vi "Report.vi"() -> ()   [LabVIEW 2017]
uses:
  <vilib>/Utility/miscctls.llb/LVRowAndColumnUnsignedTypeDef.ctl
  bcf87072-937c-4590-92ea-1cc62e0fba93.vi
  a160b8e7-0040-4e34-a052-5f80b3aab475.vi
  <vilib>/Array/Sort 2D Array - Pop Stack.vi
  <vilib>/Array/Sort 2D Array - Push Stack.vi
  <vilib>/addons/database/Connection.llb/DB Tools Open Connec (String).vi
  <vilib>/Utility/file.llb/Write Delimited Spreadsheet (string).vi
  Global/Global 1.vi
  <vilib>/regexp/Match Regular Expression.xnode
  <vilib>/addons/database/NI_Database_API.lvlib
  <vilib>/Utility/NIReport.llb/NI_report.lvclass
  <vilib>/Utility/NIReport.llb/Append Text Table to Report (wrap).vi
panel:
  out "reposr save header":string[](array[string])
  in  "SELECT REPORT TYPE":string(combo)="WITH TRECIABILITY"
  out "error out":errorcluster
  in  "error in (no error)":errorcluster
  in  "GET REPORT":bool
  in  "EXIT":bool
  in  "EXPORT TO EXCEL":bool
  in  "TO":timestamp format="%<%x>T"
  in  "FROM":timestamp format="%<%x>T"
  in  "BARCODE":string
  in  "TYPE":string(combo)="DATE TIME"
  in  "STATION WISE":string(combo)="0"
  out "Table":string[][](table)
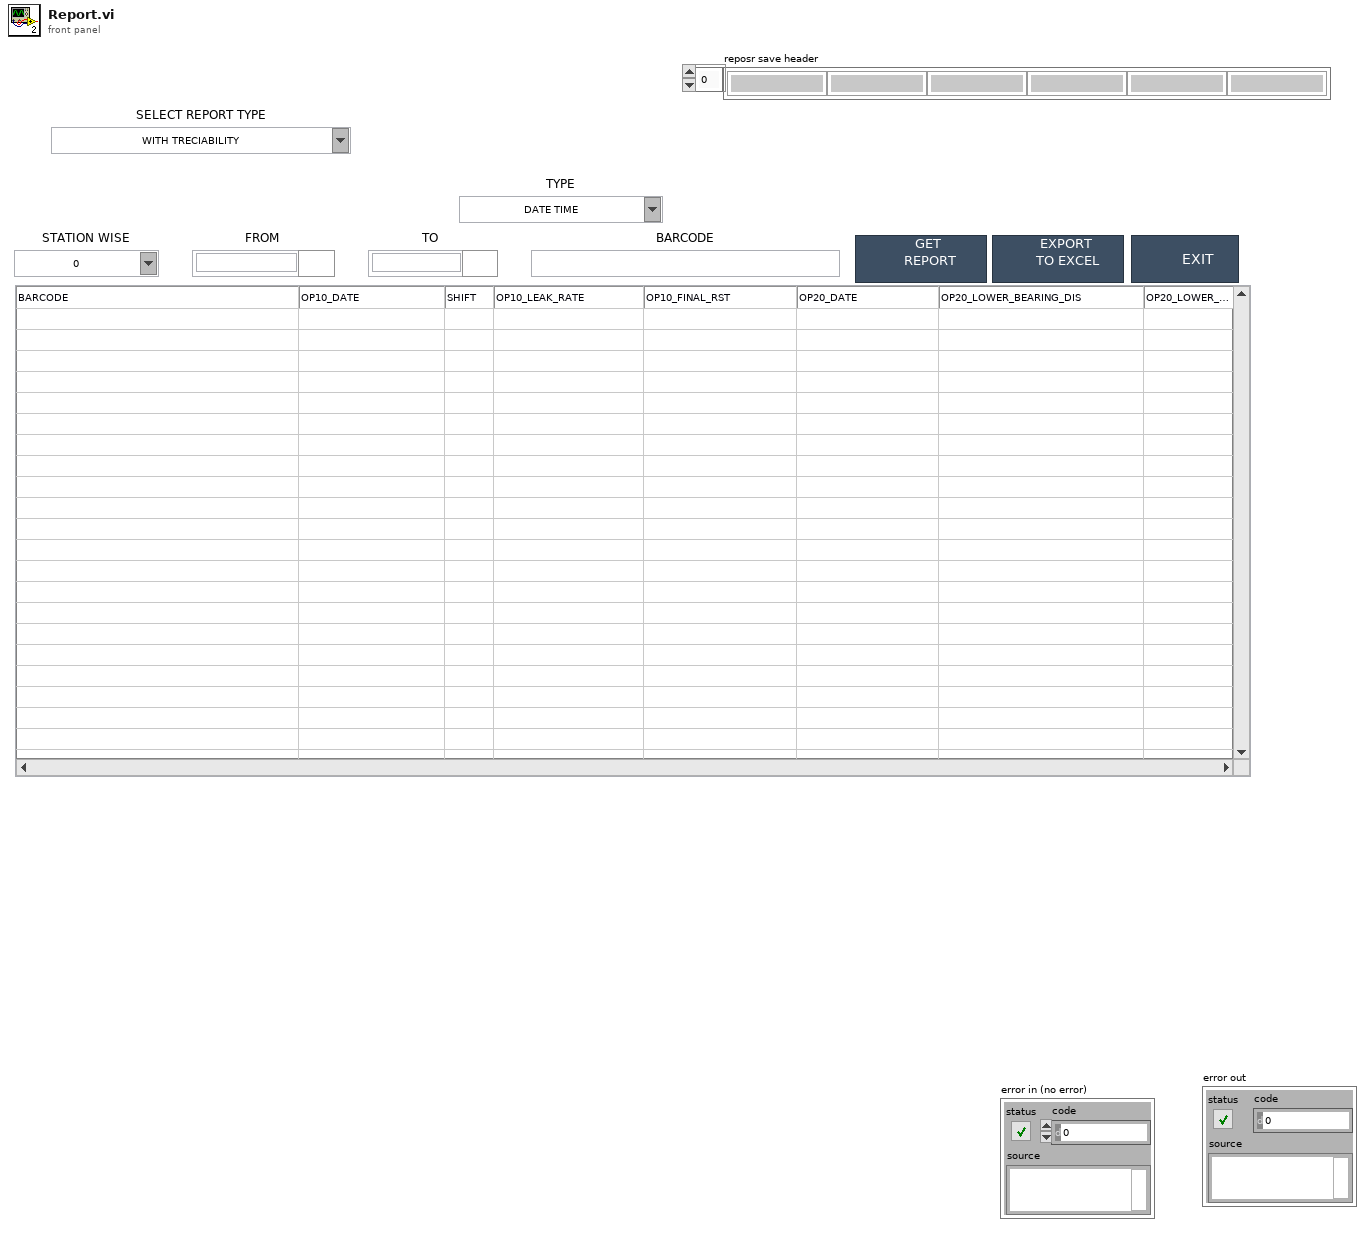
[diagram p1: front panel]
types:
  T1 = typedef "NI_Database_API.lvlib/Conn ObjectReference.ctl" = refnum<k1>
  T2 = typedef "LVRowAndColumnUnsignedTypeDef.ctl" = cluster{"Row":u32, "Column":u32}
  T3 = enum16{"Standard Report", "HTML", "Word", "Excel"}
  T4 = enum16{"maximized", "minimized", "normal", "no change"}
  T5 = typedef "LVRowAndColumnTypeDef.ctl" = cluster{"Row":i32, "Column":i32}
  T6 = enum32{"invalid app kind", "Development System", "Run Time System", "Student Edition", "Embedded LabVIEW", "Evaluation", "Custom"}
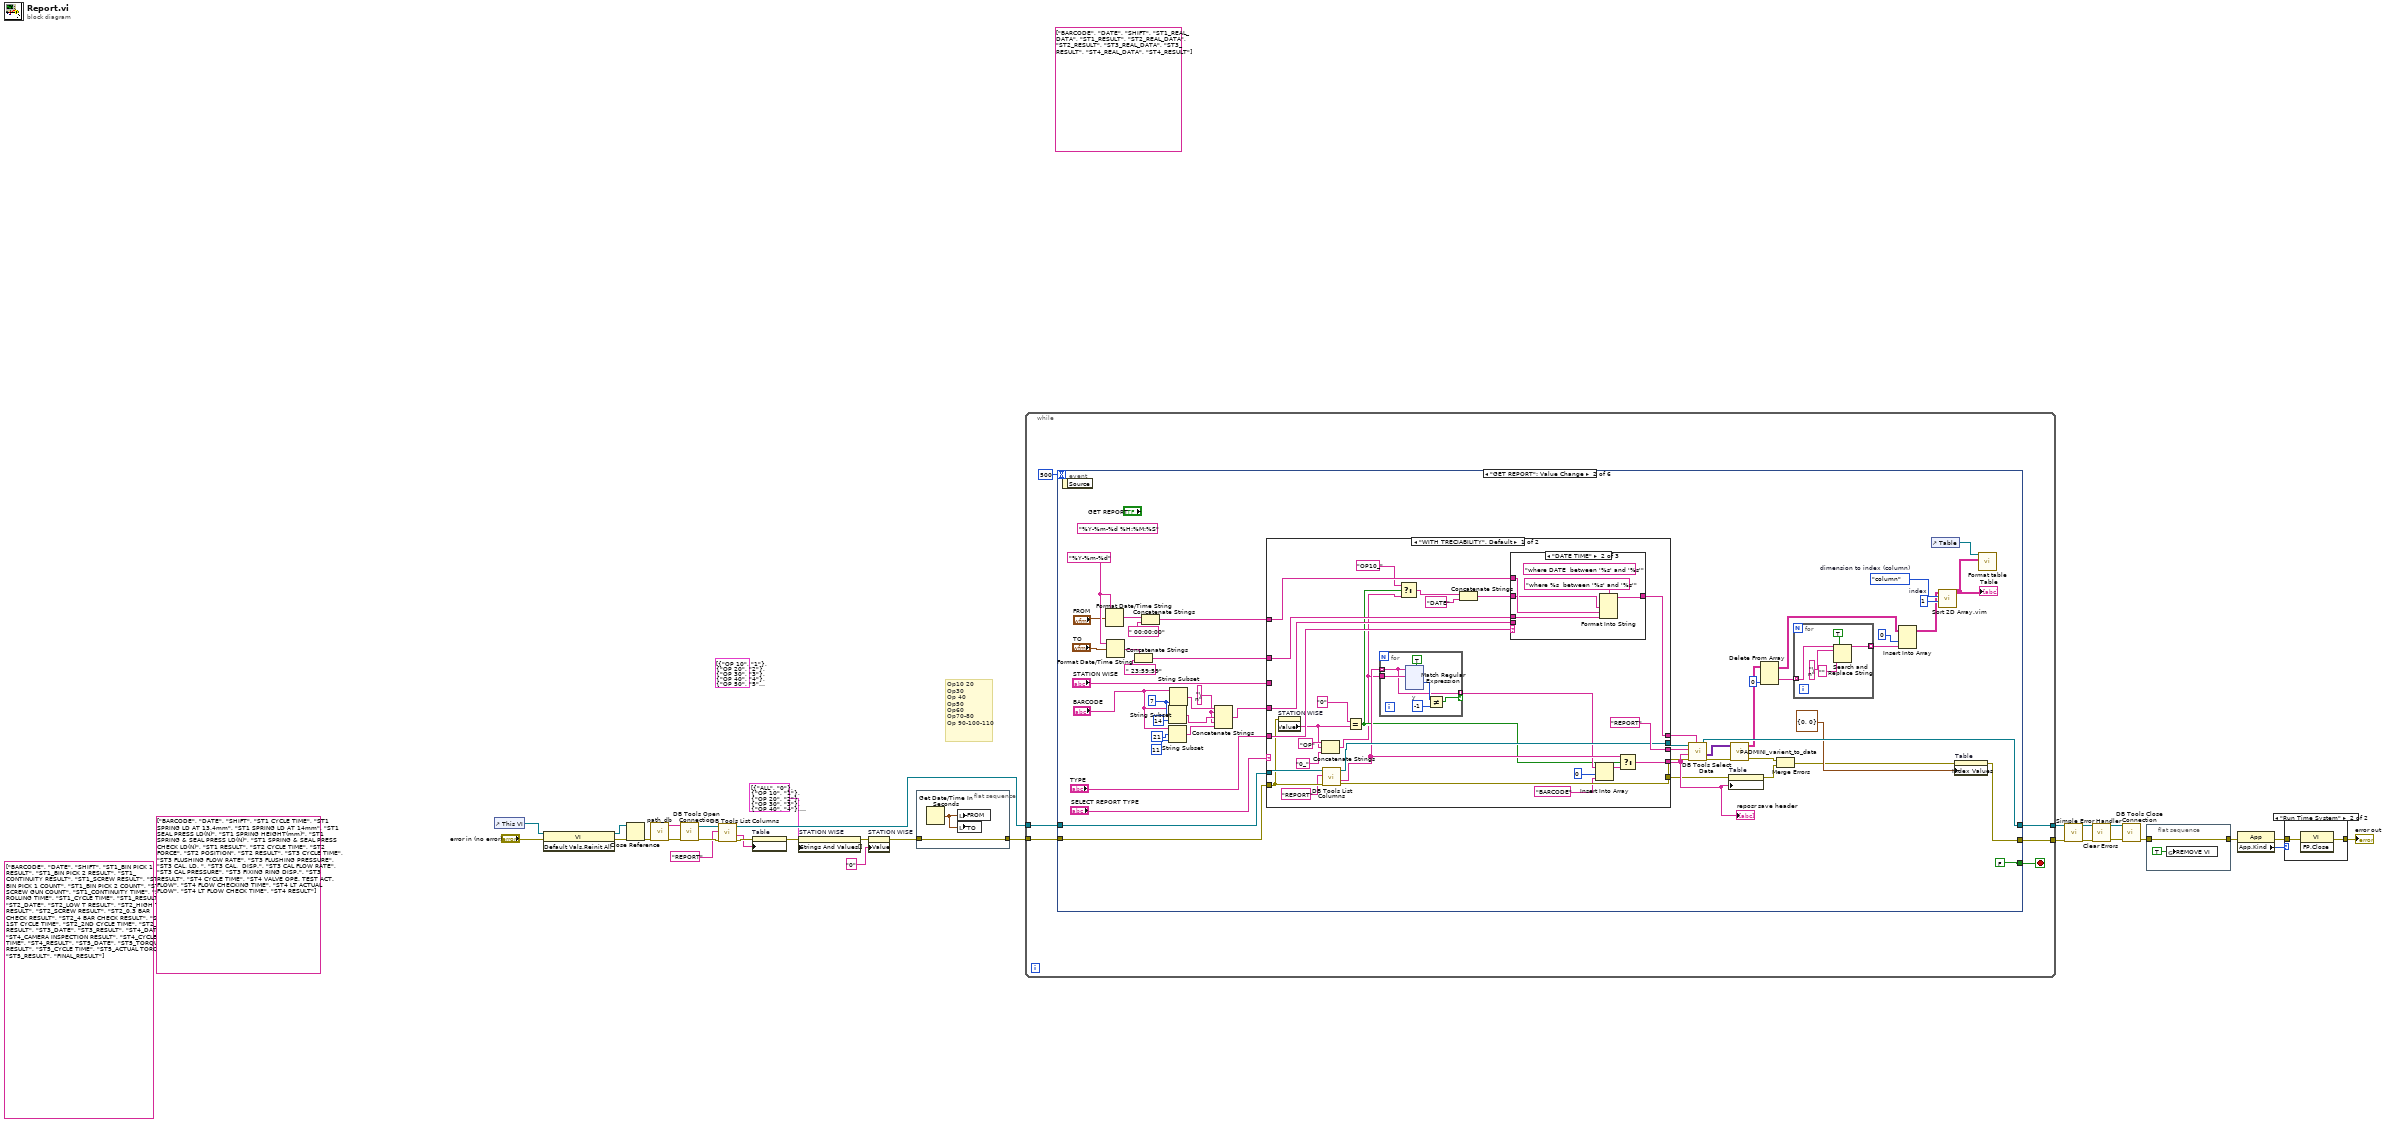
[diagram p0: block diagram]
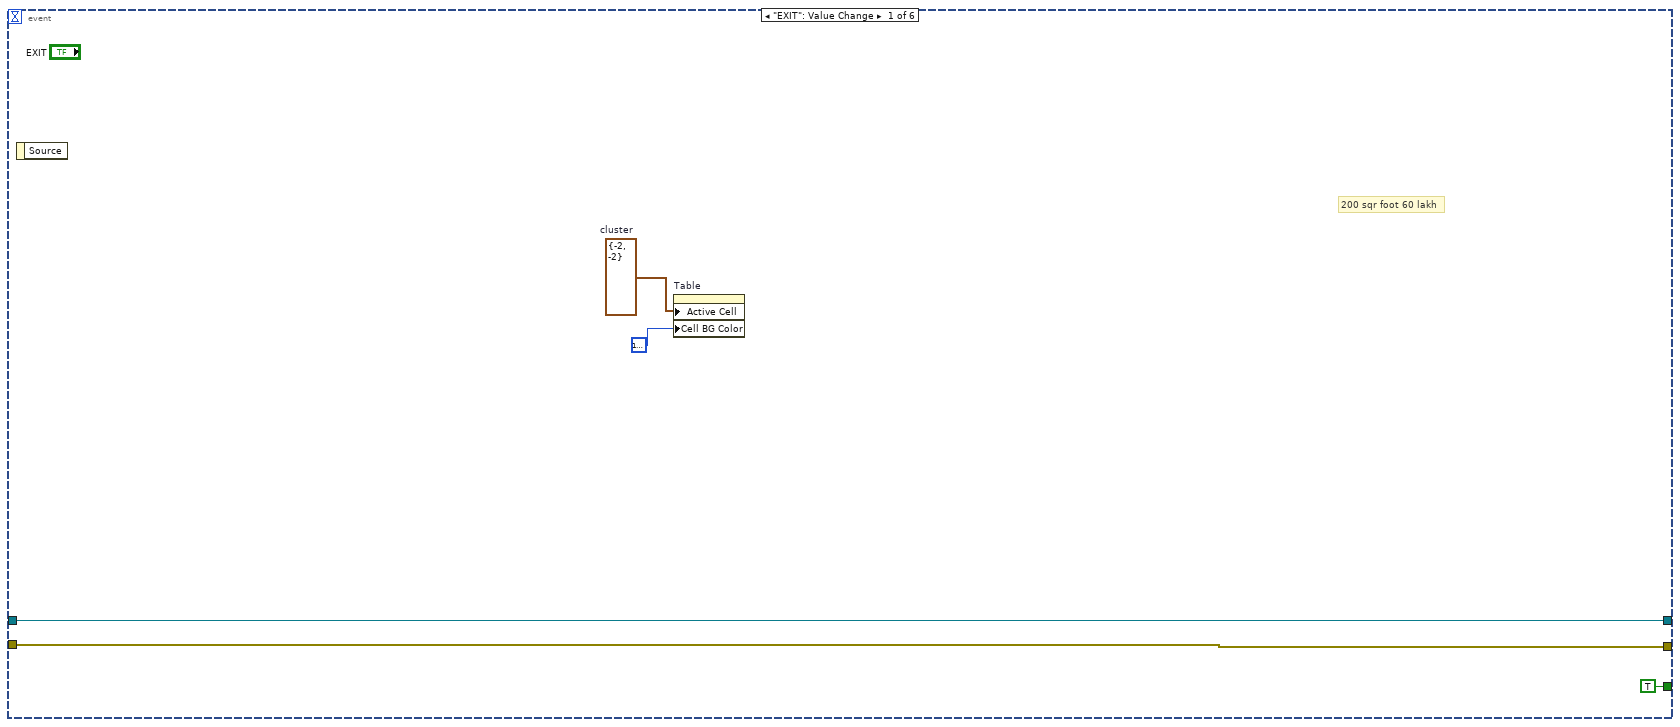
[diagram p2: hidden frame]
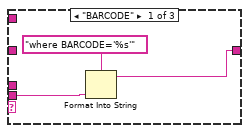
[diagram p3: hidden frame]
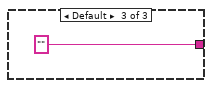
[diagram p4: hidden frame]
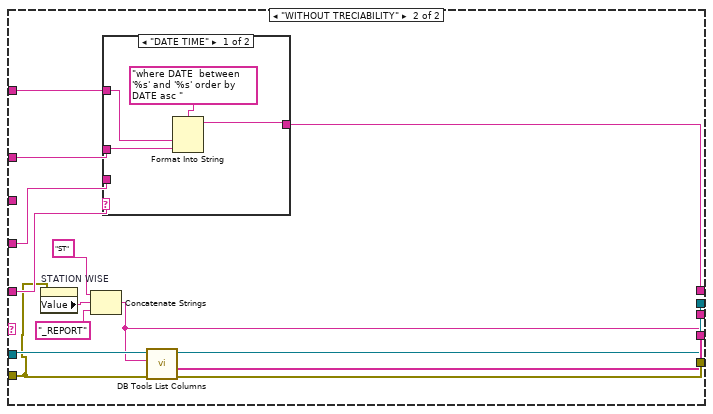
[diagram p5: hidden frame]
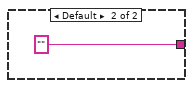
[diagram p6: hidden frame]
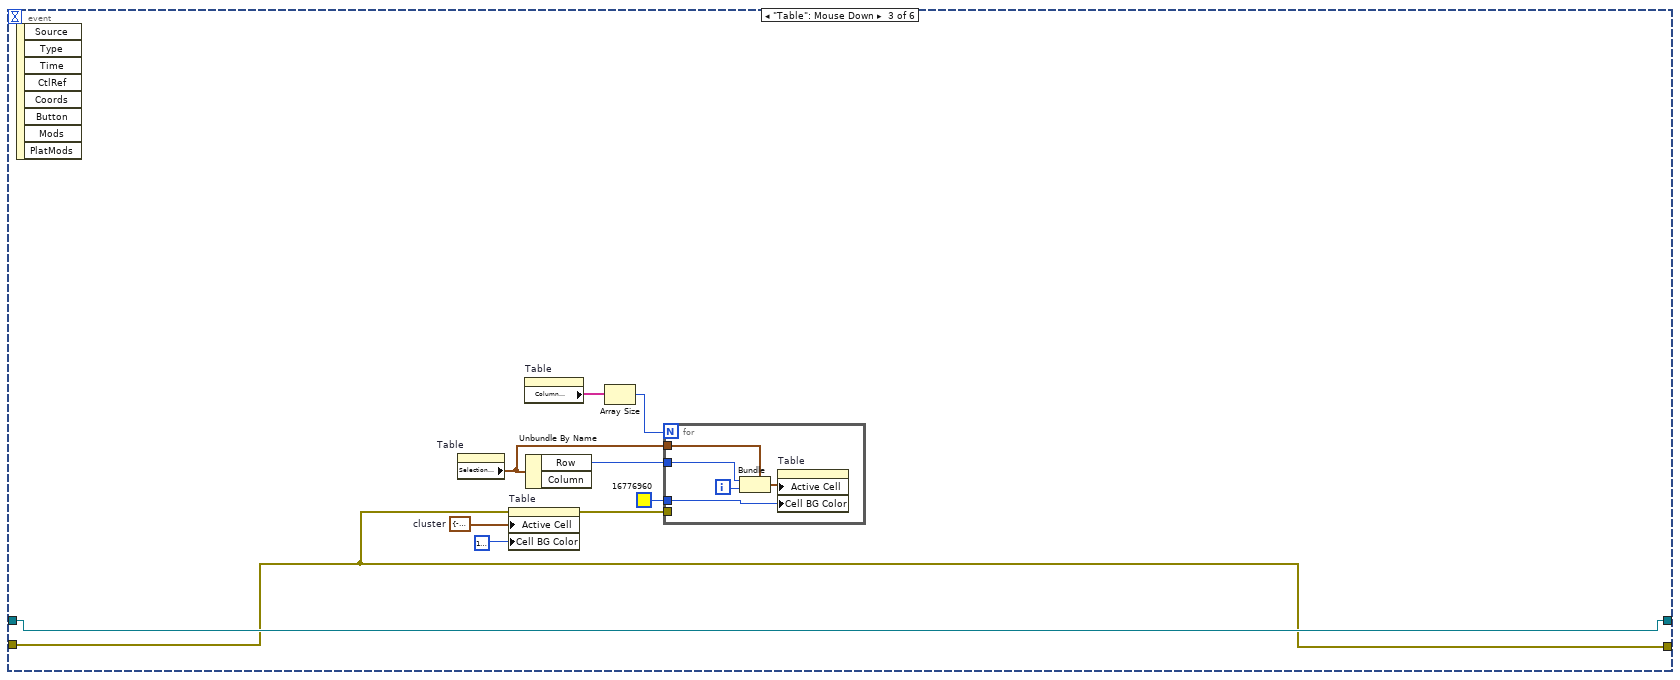
[diagram p7: hidden frame]
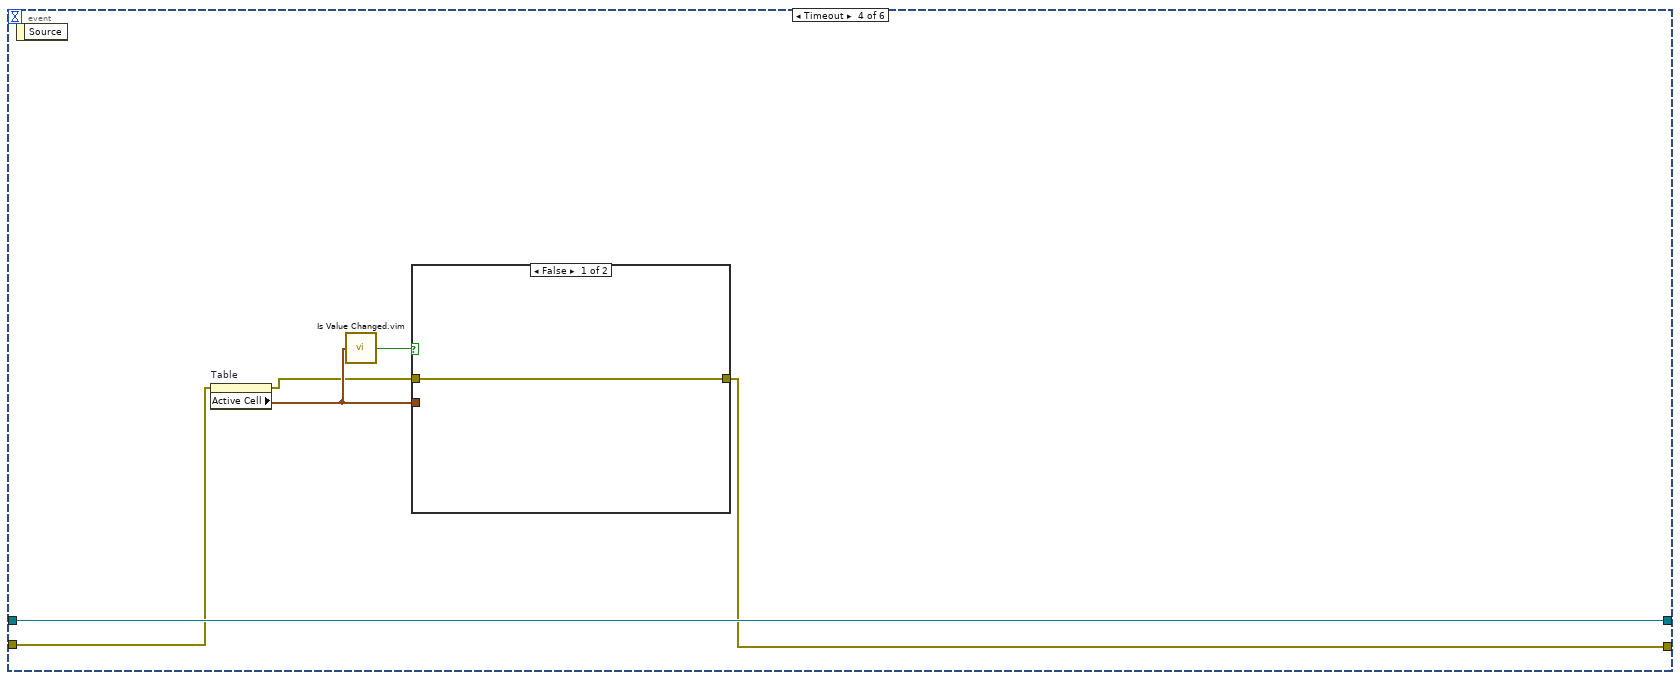
[diagram p8: hidden frame]
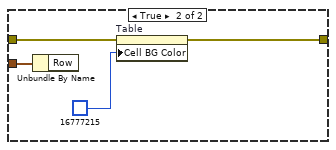
[diagram p9: hidden frame]
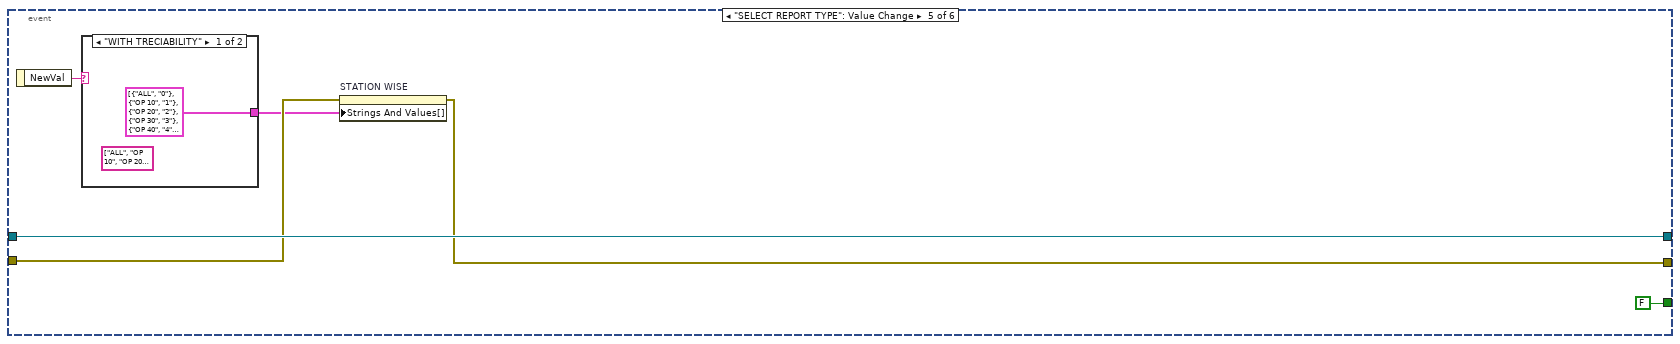
[diagram p10: hidden frame]
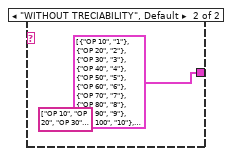
[diagram p11: hidden frame]
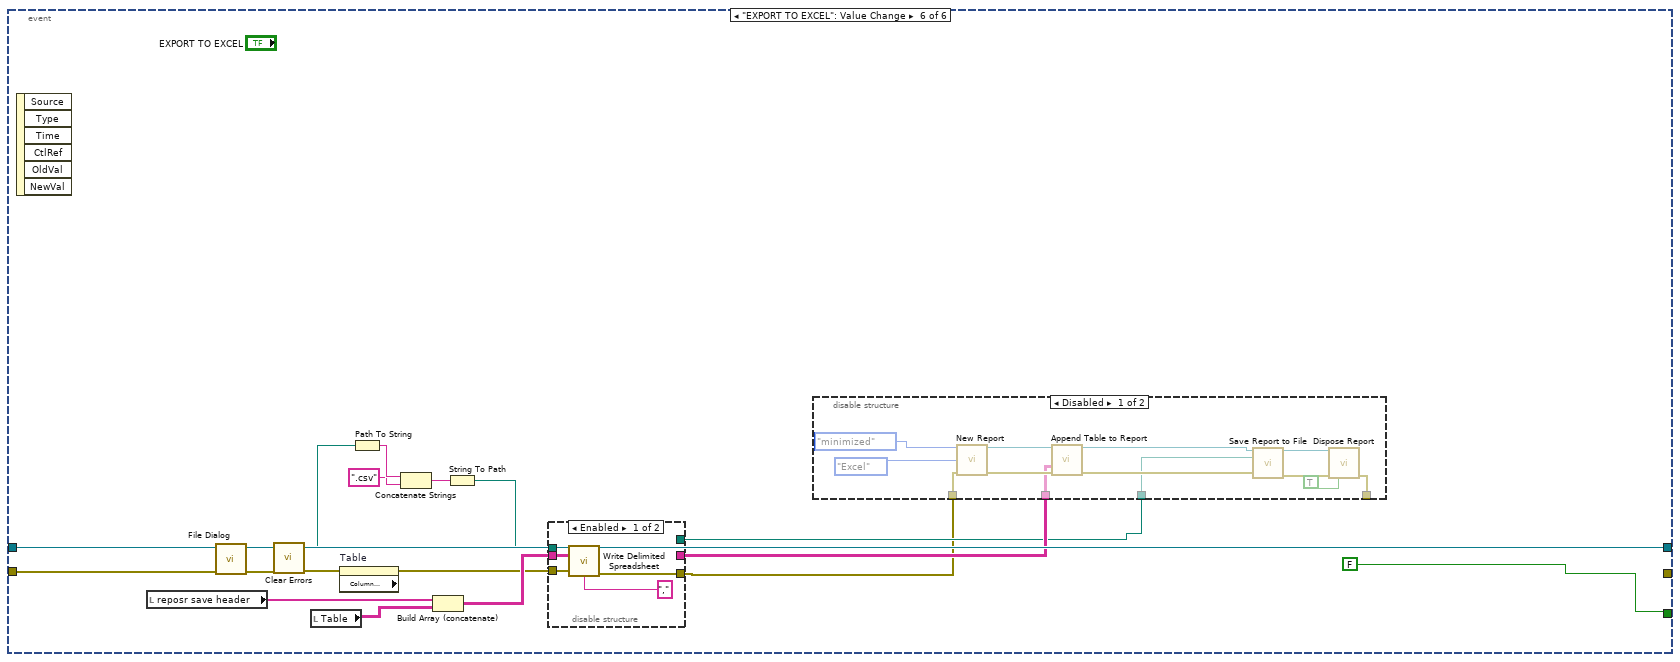
[diagram p12: hidden frame]
diagram:
  (unwired) cluster{"String":string, "Value":string}[] [{"String"="OP 10", "Value"="1"}, {"String"="OP 20", "Value"="2"}, {"String"="OP 30", "Value"="3"}, {"String"="OP 40", "Value"="4"}, {"String"="OP 50", "Value"="5"}, {"String"="OP 60", "Value"="6"}, {"String"="OP 70", "Value"="7"}, {"String"="OP 80", "Value"="8"}, {"String"="OP 90", "Value"="9"}, {"String"="OP 100", "Value"="10"}, {"String"="OP 110", "Value"="11"}] ("Strings And Values [] 2")
  (unwired) string[] ["BARCODE", "DATE", "SHIFT", "ST1_REAL_DATA", "ST1_RESULT", "ST2_REAL_DATA", "ST2_RESULT", "ST3_REAL_DATA", "ST3_RESULT", "ST4_REAL_DATA", "ST4_RESULT"]
  (unwired) string[] ["BARCODE", "DATE", "SHIFT", "ST1_BIN PICK 1 RESULT", "ST1_BIN PICK 2 RESULT", "ST1_CONTINUITY RESULT", "ST1_SCREW RESULT", "ST1_BIN PICK 1 COUNT", "ST1_BIN PICK 2 COUNT", "ST1_SCREW GUN COUNT", "ST1_CONTINUITY TIME", "ST1_ROLLING TIME", "ST1_CYCLE TIME", "ST1_RESULT", "ST2_DATE", "ST2_LOW T RESULT", "ST2_HIGH T RESULT", "ST2_SCREW RESULT", "ST2_0.3 BAR CHECK RESULT", "ST2_4 BAR CHECK RESULT", "ST2_1ST CYCLE TIME", "ST2_2ND CYCLE TIME", "ST2_RESULT", "ST3_DATE", "ST3_RESULT", "ST4_DATE", "ST4_CAMERA INSPECTION RESULT", "ST4_CYCLE TIME", "ST4_RESULT", "ST5_DATE", "ST5_TORQUE RESULT", "ST5_CYCLE TIME", "ST5_ACTUAL TORQUE", "ST5_RESULT", "FINAL_RESULT"]
  (unwired) string[] ["BARCODE", "DATE", "SHIFT", "ST1 CYCLE TIME", "ST1 SPRING LD AT 13.4mm", "ST1 SPRING LD AT 14mm", "ST1 SEAL PRESS LD(N)", "ST1 SPRING HEIGHT(mm)", "ST1 SPRING & SEAL PRESS LD(N)", "ST1 SPRING & SEAL PRESS CHECK LD(N)", "ST1 RESULT", "ST2 CYCLE TIME", "ST2 FORCE", "ST2 POSITION", "ST2 RESULT", "ST3 CYCLE TIME", "ST3 FLUSHING FLOW RATE", "ST3 FLUSHING PRESSURE", "ST3 CAL. LD. ", "ST3 CAL.  DISP.", "ST3 CAL FLOW RATE", "ST3 CAL PRESSURE", "ST3 FIXING RING DISP.", "ST3 RESULT", "ST4 CYCLE TIME", "ST4 VALVE OPE. TEST ACT. FLOW", "ST4 FLOW CHECKING TIME", "ST4 LT ACTUAL FLOW", "ST4 LT FLOW CHECK TIME", "ST4 RESULT"]
  # "Op10 20\nOp30\nOp 40\nOp50\nOp60\nOp70-80\nOp 90-100-110"
  n1 = control-ref of="This VI"() -> (w28:refnum<vi>)
  n2 = invoke class="VI" method="Default Vals.Reinit All"(reference=w28, error in="error in (no error)") -> (reference out=w26:refnum<vi>, error out=w25:errorcluster)  [unwired: 1 in, 1 out]
  n3 = Close Reference(reference=w26, error in (no error)=w25) -> (error out=w16:errorcluster)
  n4 = call "path_db.vi"("error in"=w16) -> ("error out"=w18:errorcluster, "resulting string"=w17:string)  [unwired: 9 in]
  n5 = call-poly <vilib>:"DB Tools Open Connection.vi"("error in (no error)"=w18, "connection information"=w17) -> ("error out"=w11:errorcluster, "connection reference"=w8:T1)  [unwired: 6 in]
  n6 = call <vilib>:"DB Tools List Columns.vi"("error in (no error)"=w11, "table"="REPORT", "connection reference"=w8) -> ("error out"=w10:errorcluster, "columns"=w7:string[], "connection reference out"=w9:T1)  [unwired: 1 in, 1 out]
  n7 = property on="Table" class="Tbl (strict)"(error in=w10, "Column Headers[]"=w7) -> (error out=w13:errorcluster)  [unwired: 1 in, 1 out]
  n8 = property on="STATION WISE" class="CmbBox"(error in=w13, "Strings And Values[]"=cluster{"String":string, "Value":string}[] [{"String"="ALL", "Value"="0"}, {"String"="OP 10", "Value"="1"}, {"String"="OP 20", "Value"="2"}, {"String"="OP 30", "Value"="3"}, {"String"="OP 40", "Value"="4"}, {"String"="OP 50", "Value"="5"}, {"String"="OP 60", "Value"="6"}, {"String"="OP 70", "Value"="7"}, {"String"="OP 80", "Value"="8"}, {"String"="OP 90", "Value"="9"}, {"String"="OP 100", "Value"="10"}, {"String"="OP 110", "Value"="11"}] ("Strings And Values [] 2")) -> (error out=w5:errorcluster)  [unwired: 1 in, 1 out]
  n9 = property on="STATION WISE" class="CmbBox"(error in=w5, "Value"="0") -> (error out=w4:errorcluster)  [unwired: 1 in, 1 out]
  n10 = flat-sequence {
    tunnel: w4 -> [w29]
    tunnel: [w29] -> w12
    frame #0 {
      n11 = Get Date/Time In Seconds() -> (seconds since 1Jan1904=w30:timestamp)
      n12 = local write "FROM"(w30) -> ()
      n13 = local write "TO"(w30) -> ()
    }
  }
  n14 = while {
    tunnel: [w33] -> w1
    tunnel: w12 -> [w35]
    tunnel: w9 -> [w34]
    tunnel: [w32] -> w14
    stop <- w36 stop-if-true
    n15 = event shown="[1] \"GET REPORT\": Value Change" {
      selector: _ -> [_ _ _ _ _ _]
      dyn-events: _ -> [_ _ _ _ _ _]
      timeout: 500 -> [_ _ _ _ _ _]
      tunnel: [TRUE FALSE _ _ FALSE FALSE] -> w36
      tunnel: w35 -> [w39 w70 w279 w288 w300 w309]
      tunnel: w34 -> [w40 w68 w280 w291 w302 w320]
      tunnel: [w40 w76 w280 w291 w302 w320] -> w32
      tunnel: [w39 w58 w279 w286 w297 _] -> w33
      event "EXIT": Value Change {
        w37 = cluster{"Row":i32, "Row":i32} {"Row"=-2, "Row"=-2}  # cluster
        # "200 sqr foot 60 lakh"
        n16 = event-data() -> ()  [unwired: 1 in, 1 out]
        n17 = property on="Table" class="Tbl (strict)"("Active Cell"=w37, "Cell BG Color"=u32 16777226) -> ()  [unwired: 2 in, 2 out]
      }
      event "GET REPORT": Value Change {
        w46 = 1  # index
        w47 = enum16{"column", "row"}."column"  # dimension to index (column)
        w50 = "\n"
        w57 = 7 ("line index")
        (unwired) "%Y-%m-%d %H:%M:%S" ("time format string (%c)")
        w88 = "%Y-%m-%d" ("time format string (%c)")
        n18 = event-data() -> ()  [unwired: 1 in, 1 out]
        n19 = Format Date/Time String(time format string (%c)=w88, seconds (now)="FROM") -> (date/time string=w82:string)  [unwired: 1 in]
        n20 = Format Date/Time String(time format string (%c)=w88, seconds (now)="TO") -> (date/time string=w79:string)  [unwired: 1 in]
        n21 = Concatenate Strings(w79, " 23:59:59" ("time format string (%c)")) -> (w78:string)
        n22 = Concatenate Strings(w82, " 00:00:00" ("time format string (%c)")) -> (w81:string)
        n23 = String Subset(string="BARCODE", offset (0)=w57, length (rest)=14 ("line index")) -> (substring=w52:string)
        n24 = String Subset(string="BARCODE", offset (0)=21 ("line index"), length (rest)=11 ("line index")) -> (substring=w51:string)
        n25 = String Subset(string="BARCODE", length (rest)=w57) -> (substring=w53:string)  [unwired: 1 in]
        n26 = Concatenate Strings(w53, w50, w52, w50, w51) -> (w49:string)
        n27 = case shown="\"WITH TRECIABILITY\", Default" "SELECT REPORT TYPE" {
          tunnel: "TYPE" -> [w122 w265]
          tunnel: [w121 w264] -> w89
          tunnel: w49 -> [w120 w263]
          tunnel: w81 -> [w119 w262]
          tunnel: w78 -> [w104 w258]
          tunnel: "STATION WISE" -> [_ _]
          tunnel: ["REPORT" w253] -> w71
          tunnel: w70 -> [w110 w252]
          tunnel: [w115 w257] -> w65
          tunnel: [w102 w256] -> w69
          tunnel: w68 -> [w117 w255]
          tunnel: [w116 w254] -> w67
          frame "WITH TRECIABILITY", Default {
            n28 = property on="STATION WISE" class="CmbBox"(error in=w110) -> ("Value"=w105:string)  [unwired: 1 in, 2 out]
            n29 = Concatenate Strings("OP" ("element"), w105, "0_" ("element")) -> (w97:string)
            n30 = call <vilib>:"DB Tools List Columns.vi"("error in (no error)"=w110, "table"="REPORT", "connection reference"=w117) -> ("error out"=w115:errorcluster, "columns"=w109:string[], "connection reference out"=w116:T1)  [unwired: 1 in, 1 out]
            n31 = Equal?(x="0", y=w105) -> (x = y?=w99:bool)
            n32 = for {
              tunnel: w109 -> [w124] mode=indexing
              tunnel: w97 -> [w128]
              tunnel: [w124] -> w103 mode=indexing if=w123
              w125 = -1  # y
              n33 = xnode "Match Regular Expression"("input string"=w124, "regular expression"=w128, "multiline? (F)"=TRUE) -> ("offset past match"=w126:i32)  [unwired: 3 in, 4 out]
              n34 = Not Equal?(x=w126, y=w125) -> (x != y?=w123:bool)
            }
            n35 = Select(t="OP10_", s=w99, f=w97) -> (s? t:f=w96:string)
            n36 = Concatenate Strings(w96, "DATE") -> (w100:string)
            n37 = case shown="\"DATE TIME\"" w122 {
              tunnel: [w244 w249 ""] -> w121
              tunnel: w120 -> [w243 _ _]
              tunnel: w119 -> [_ w248 _]
              tunnel: w104 -> [_ w247 _]
              tunnel: w100 -> [_ w246 _]
              frame "BARCODE" {
                n38 = Format Into String(format string="where BARCODE='%s'", w243) -> (resulting string=w244:string)  [unwired: 2 in, 1 out]
              }
              frame "DATE TIME" {
                (unwired) "where DATE  between '%s' and '%s'"
                n39 = Format Into String(format string="where %s  between '%s' and '%s'", w246, w248, w247) -> (resulting string=w249:string)  [unwired: 2 in, 1 out]
              }
              frame Default {
              }
            }
            n40 = Insert Into Array(array=w103, index=0, new element="BARCODE" ("String")) -> (w113:string[])
            n41 = Select(t=w109, s=w99, f=w113) -> (s? t:f=w102:string[])
          }
          frame "WITHOUT TRECIABILITY" {
            n42 = property on="STATION WISE" class="CmbBox"(error in=w252) -> ("Value"=w261:string)  [unwired: 1 in, 2 out]
            n43 = Concatenate Strings("ST", w261, "_REPORT") -> (w253:string)
            n44 = case shown="\"DATE TIME\"" w265 {
              tunnel: [w269 ""] -> w264
              tunnel: w263 -> [_ _]
              tunnel: w262 -> [w268 _]
              tunnel: w258 -> [w267 _]
              frame "DATE TIME" {
                n45 = Format Into String(format string="where DATE  between '%s' and '%s' order by DATE asc ", w268, w267) -> (resulting string=w269:string)  [unwired: 2 in, 1 out]
              }
              frame Default {
              }
            }
            n46 = call <vilib>:"DB Tools List Columns.vi"("error in (no error)"=w252, "table"=w253, "connection reference"=w255) -> ("error out"=w257:errorcluster, "columns"=w256:string[], "connection reference out"=w254:T1)  [unwired: 1 in, 1 out]
          }
        }
        "reposr save header" <- w69
        n47 = call <vilib>:"DB Tools Select Data.vi"("condition"=w89, "error in (no error)"=w65, "columns"=w69, "table"=w71, "connection reference"=w67) -> ("error out"=w74:errorcluster, "data"=w77:variant[][], "connection reference out"=w76:T1)  [unwired: 1 in]
        n48 = property on="Table" class="Tbl (strict)"(error in=w65, "Column Headers[]"=w69) -> (error out=w73:errorcluster)  [unwired: 1 in, 1 out]
        n49 = call "PADMINI_varient_to_data.vi"("error in (no error)"=w74, "data"=w77) -> ("error out"=w72:errorcluster, "Array"=w60:string[][])  [unwired: 8 in]
        n50 = Delete From Array(array=w60, index (col)=0 ("disabled index (col)")) -> (deleted portion=w63:string[], array with subset deleted=w61:string[][])  [unwired: 2 in]
        n51 = Merge Errors(w72, w73) -> (w42:errorcluster)
        n52 = for {
          tunnel: w63 -> [w92] mode=indexing
          tunnel: [w91] -> w62 mode=indexing
          n53 = Search and Replace String(replace all?=TRUE ("replace all? (F)"), input string=w92, search string="\n", replace string="" ("replace string (\"\")")) -> (result string=w91:string)  [unwired: 4 in, 3 out]
        }
        n54 = Insert Into Array(array=w61, index (col)=0 ("disabled index (col)"), new element=w62) -> (w45:string[][])  [unwired: 1 in]
        n55 = control-ref of="Table"() -> (w44:refnum<vi>)
        n56 = call "Sort 2D Array.vim"("index"=w46, "dimension to index (column)"=w47, "2D array"=w45) -> ("sorted 2D array"=w43:string[][])  [unwired: 7 in, 1 out]
        "Table" <- w43
        n57 = property on="Table" class="Tbl (strict)"(error in=w42, "Index Values"=T2 {"Row"=0, "Column"=0}) -> (error out=w58:errorcluster)  [unwired: 1 in, 1 out]
        n58 = call "Format table.vi"("Table Control"=w43, "reference"=w44) -> ()  [unwired: 7 in, 1 out]
      }
      event "Table": Mouse Down {
        w274 = cluster{"Row":i32, "Row":i32} {"Row"=-2, "Row"=-2}  # cluster
        n59 = event-data() -> ()  [unwired: 1 in, 8 out]
        n60 = property on="Table" class="Tbl (strict)"() -> ("Selection Start"=w276:T5)  [unwired: 2 in, 2 out]
        n61 = property on="Table" class="Tbl (strict)"(error in=w279, "Active Cell"=w274, "Cell BG Color"=u32 16777226) -> (error out=w275:errorcluster)  [unwired: 1 in, 1 out]
        n62 = property on="Table" class="Tbl (strict)"() -> ("Column Headers[]"=w272:string[])  [unwired: 2 in, 2 out]
        n63 = Unbundle By Name(w276) -> ("Row"=w278:i32)  [unwired: 1 out]
        n64 = Array Size(array=w272) -> (size(s)=w271:i32)
        n65 = for {
          N: w271 -> [_]
          tunnel: u32 16776960 -> [w285]
          tunnel: w276 -> [w284]
          tunnel: w278 -> [w283]
          tunnel: w275 -> [_]
          i -> [w282]
          n66 = Bundle(cluster=w284, "Row"=w283, "Column"=w282) -> (w281:T5)
          n67 = property on="Table" class="Tbl (strict)"("Active Cell"=w281, "Cell BG Color"=w285) -> ()  [unwired: 2 in, 2 out]
        }
      }
      event Timeout {
        n68 = event-data() -> ()  [unwired: 1 in, 1 out]
        n69 = property on="Table" class="Tbl (strict)"(error in=w288) -> (error out=w287:errorcluster, "Active Cell"=w290:T5)  [unwired: 1 in, 1 out]
        n70 = call "Is Value Changed.vim"("value"=w290) -> ("changed or first call?"=w289:bool)
        n71 = case shown="False" w289 {
          tunnel: w290 -> [_ w296]
          tunnel: w287 -> [w292 w294]
          tunnel: [w292 w293] -> w286
          frame False {
          }
          frame True {
            n72 = Unbundle By Name(w296) -> ()  [unwired: 1 out]
            n73 = property on="Table" class="Tbl (strict)"(error in=w294, "Cell BG Color"=u32 16777215) -> (error out=w293:errorcluster)  [unwired: 1 in, 1 out]
          }
        }
      }
      event "SELECT REPORT TYPE": Value Change {
        n74 = event-data() -> ("NewVal"=w301:string)  [unwired: 1 in]
        n75 = case shown="\"WITH TRECIABILITY\"" w301 {
          tunnel: [cluster{"String":string, "Value":string}[] [{"String"="ALL", "Value"="0"}, {"String"="OP 10", "Value"="1"}, {"String"="OP 20", "Value"="2"}, {"String"="OP 30", "Value"="3"}, {"String"="OP 40", "Value"="4"}, {"String"="OP 50", "Value"="5"}, {"String"="OP 60", "Value"="6"}, {"String"="OP 70", "Value"="7"}, {"String"="OP 80", "Value"="8"}, {"String"="OP 90", "Value"="9"}, {"String"="OP 100", "Value"="10"}, {"String"="OP 110", "Value"="11"}] ("Strings And Values [] 2") cluster{"String":string, "Value":string}[] [{"String"="OP 10", "Value"="1"}, {"String"="OP 20", "Value"="2"}, {"String"="OP 30", "Value"="3"}, {"String"="OP 40", "Value"="4"}, {"String"="OP 50", "Value"="5"}, {"String"="OP 60", "Value"="6"}, {"String"="OP 70", "Value"="7"}, {"String"="OP 80", "Value"="8"}, {"String"="OP 90", "Value"="9"}, {"String"="OP 100", "Value"="10"}, {"String"="OP 110", "Value"="11"}] ("Strings And Values [] 2")] -> w298
          frame "WITH TRECIABILITY" {
            (unwired) string[] ["ALL", "OP 10", "OP 20", "OP 30", "OP 40", "OP 50", "OP 60", "OP 70", "OP 80", "OP 90", "OP 100", "OP 110"] ("Strings []")
          }
          frame "WITHOUT TRECIABILITY", Default {
            (unwired) string[] ["OP 10", "OP 20", "OP 30", "OP 40", "OP 50", "OP 60", "OP 70", "OP 80", "OP 90", "OP 100", "OP 110"] ("Strings []")
          }
        }
        n76 = property on="STATION WISE" class="CmbBox"(error in=w300, "Strings And Values[]"=w298) -> (error out=w297:errorcluster)  [unwired: 1 in, 1 out]
      }
      event "EXPORT TO EXCEL": Value Change {
        n77 = event-data() -> ()  [unwired: 1 in, 6 out]
        n78 = local read "reposr save header"() -> (w305:string[])
        n79 = call "File Dialog"("error in"=w309) -> ("selected path"=w318:path, "error out"=w319:errorcluster)  [unwired: 11 in, 2 out]
        n80 = call <vilib>:"Clear Errors.vi"("error in (no error)"=w319) -> ("error out"=w312:errorcluster)  [unwired: 5 in, 1 out]
        n81 = local read "Table"() -> (w321:string[][])
        n82 = property on="Table" class="Tbl (strict)" props=["Column Headers[]"](error in=w312) -> (error out=w311:errorcluster)  [unwired: 1 in, 2 out]
        n83 = Path To String(path=w318) -> (string=w317:string)
        n84 = Concatenate Strings(w317, ".csv" ("string")) -> (w315:string)
        n85 = Build Array (concatenate)(w305, w321) -> (w313:string[][])
        n86 = String To Path(string=w315) -> (path=w314:path)
        n87 = disable-structure shown="Enabled" {
          disable-tunnel: w314 -> [w340 w341]
          disable-tunnel: [w339 w343] -> w306
          disable-tunnel: w313 -> [w338 w342]
          disable-tunnel: w311 -> [w336 w343]
          disable-tunnel: [_ w342] -> w308
          disable-tunnel: [_ w341] -> w307
          frame Enabled {
            n88 = call-poly <vilib>:"Write Delimited Spreadsheet.vi"("file path (dialog if empty)"=w340, "2D data"=w338, "error in (no error)"=w336, "delimiter (\\t)"="," ("delimiter (\\t)")) -> ("error out"=w339:errorcluster)  [unwired: 10 in, 1 out]
          }
          frame Disabled {
          }
        }
        n89 = disable-structure shown="Disabled" {
          disable-tunnel: w308 -> [w325 _]
          disable-tunnel: w307 -> [w324 _]
          disable-tunnel: [w323 w335] -> _
          disable-tunnel: w306 -> [w322 w335]
          frame Disabled {
            n90 = call <vilib>:"New Report.vi"("window state (normal)"=T4."minimized", "report type"=T3."Excel", "error in (no error)"=w322) -> ("report out"=w332:refnum<class "NI_report.lvclass">, "error out"=w331:errorcluster)  [unwired: 11 in]
            n91 = call-poly <vilib>:"Append Table to Report.vi"("report in"=w332, "text data"=w325, "error in (no error)"=w331) -> ("report out"=w328:refnum<class "NI_report.lvclass">, "error out"=w330:errorcluster)  [unwired: 9 in, 2 out]
            n92 = call-dynamic "Save Report to File.vi"("report in"=w328, "report file path"=w324, "error in (no error)"=w330) -> ("report out"=w327:refnum<class "NI_report.lvclass">, "error out"=w329:errorcluster)  [unwired: 11 in]
            n93 = call-dynamic "Dispose Report.vi"("report in"=w327, "error in (no error)"=w329, "close report? (T)"=TRUE) -> ("error out"=w323:errorcluster)  [unwired: 12 in]
          }
          frame Enabled {
          }
        }
      }
    }
  }
  n94 = call <vilib>:"Simple Error Handler.vi"("error in (no error)"=w1) -> ("error out"=w24:errorcluster)  [unwired: 4 in, 4 out]
  n95 = call <vilib>:"Clear Errors.vi"("error in (no error)"=w24) -> ("error out"=w23:errorcluster)  [unwired: 5 in, 1 out]
  n96 = call <vilib>:"DB Tools Close Connection.vi"("error in (no error)"=w23, "connection reference"=w14) -> ("error out"=w15:errorcluster)  [unwired: 5 in]
  n97 = flat-sequence {
    tunnel: [w345] -> w22
    tunnel: w15 -> [w345]
    frame #0 {
      n98 = global write "Global 1.vi" "REMOVE VI"(TRUE ("REMOVE VI")) -> ()
    }
  }
  n99 = property class="App"(error in=w22) -> (error out=w21:errorcluster, "App.Kind"=w20:T6)  [unwired: 1 in, 1 out]
  n100 = case shown="\"Run Time System\"" w20 {
    tunnel: w21 -> [w346 w348]
    tunnel: [w346 w347] -> w19
    frame "Development System", Default {
    }
    frame "Run Time System" {
      n101 = invoke class="VI" method="FP.Close"(error in=w348) -> (error out=w347:errorcluster)  [unwired: 2 in, 2 out]
    }
  }
  "error out" <- w19
